vi "integration2.vi"(8 "heading":dbl, 10 "dist":dbl, 11 "pos(i-1)":dbl[](array[numeric])) -> (3 "pos(i)":dbl[](array[numeric]))   [LabVIEW 2012]
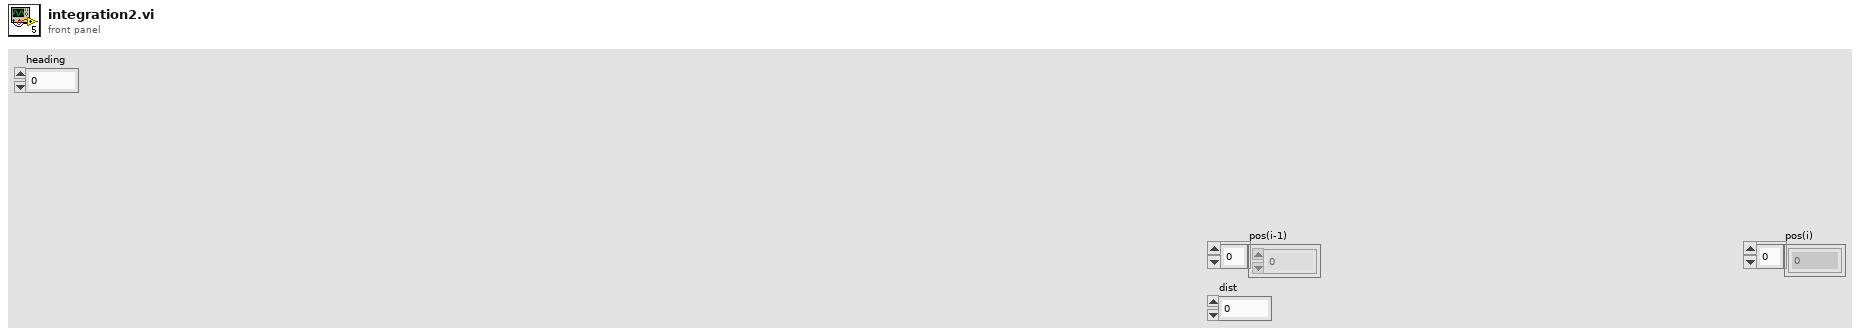
[diagram p1: front panel]
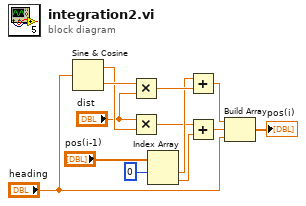
[diagram p0: block diagram]
diagram:
  n1 = Sine & Cosine(0:"heading") -> (1:w5:dbl, 2:w6:dbl)
  n2 = Multiply(x=w6, y="dist") -> (x*y=w12:dbl)
  n3 = Multiply(x="dist", y=w5) -> (x*y=w10:dbl)
  n4 = Index Array(array="pos(i-1)", index #1=0 ("index")) -> (element #1=w11:dbl, element #2=w9:dbl)  [unwired: 1 in]
  n5 = Add(x=w11, y=w12) -> (x+y=w8:dbl)
  n6 = Add(x=w10, y=w9) -> (x+y=w7:dbl)
  n7 = Build Array(w8, w7, "heading") -> (→"pos(i)":dbl[])
